vi "Get Measurement Variables from Recipe.vi"(8 "error in (no error)":errorcluster, 11 "Measurement in":refnum<class "Measurement.lvclass">) -> (0 "error out":errorcluster, 1 "Measurements":string[](array[string]), 2 "Power Measurements":string[](array[string]), 3 "Measurement Voltages":string[](array[string]))   [LabVIEW 2015, in "Measurement.lvclass"]
uses:
  Measurement.lvclass
  Test Class/Test Class.lvclass
  Classes/Application/Class/Application.lvclass
  Classes/Test Recipe/Class/Test Recipe.lvclass
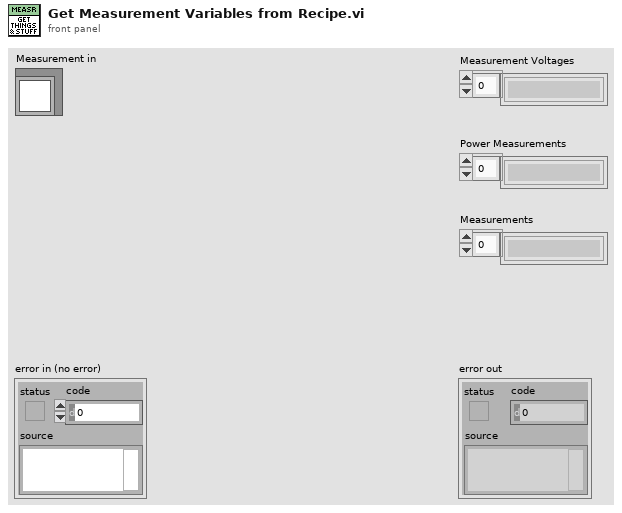
[diagram p1: front panel]
types:
  T1 = typedef "Application.lvlib/App Properties.lvclass/Class Properties -- Cluster.ctl" = cluster{"UUT Info":T2[], "Test Information":refnum<vi>, "Test Complete Event":refnum<user-event>, "Shop Floor System":refnum<class "Shop Floor System.lvclass">, "Gold Board":refnum<class "Golden Board.lvclass">, "Test Recipe":refnum<class "Test Recipe.lvclass">, "Instruments":refnum<class "Instrument.lvclass">[], "Mode":T3, "Test Results":cluster{"Pass":bool[], "Fail Codes":string[]}, "Station Config":refnum<class "Station Config.lvclass">}
  T2 = typedef "Application.lvlib/App Properties.lvclass/UUT Reference -- Cluster.ctl" = cluster{"Serial Number Reference":refnum<vi>, "Status Message Reference":refnum<vi>}
  T3 = typedef "Application.lvlib/Application.lvclass/Op Mode -- Enum.ctl" = u16
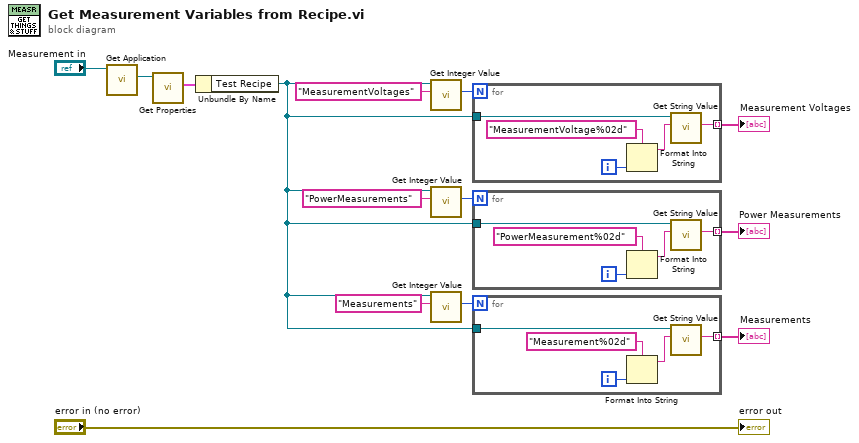
[diagram p0: block diagram]
diagram:
  n1 = call "Get Application.vi"("Test Class in"="Measurement in") -> ("Application.lvlib:Application.lvclass"=w12:refnum<class "Application.lvclass">)  [unwired: 9 in, 1 out]
  n2 = call "Get Properties.vi"("Acrobat Template in"=w12) -> ("Class Properties"=w11:T1)  [unwired: 8 in, 2 out]
  n3 = Unbundle By Name(w11) -> ("Test Recipe"=w2:refnum<class "Test Recipe.lvclass">)
  n4 = call "Get Integer Value.vi"("Name"="MeasurementVoltages", "Test Recipe in"=w2) -> ("Value"=w9:i32)  [unwired: 6 in, 3 out]
  n5 = call "Get Integer Value.vi"("Name"="PowerMeasurements", "Test Recipe in"=w2) -> ("Value"=w3:i32)  [unwired: 6 in, 3 out]
  n6 = call "Get Integer Value.vi"("Name"="Measurements", "Test Recipe in"=w2) -> ("Value"=w8:i32)  [unwired: 6 in, 3 out]
  n7 = for {
    N: w9 -> [_]
    tunnel: w2 -> [w19]
    tunnel: [w15] -> w6 mode=indexing
    i -> [w18]
    n8 = Format Into String(format string="MeasurementVoltage%02d", w18) -> (resulting string=w16:string)  [unwired: 2 in, 1 out]
    n9 = call "Get String Value.vi"("Name"=w16, "Test Recipe in"=w19) -> ("Value"=w15:string)  [unwired: 6 in, 3 out]
  }
  "Measurement Voltages" <- w6
  n10 = for {
    N: w3 -> [_]
    tunnel: w2 -> [w24]
    tunnel: [w20] -> w1 mode=indexing
    i -> [w23]
    n11 = Format Into String(format string="PowerMeasurement%02d", w23) -> (resulting string=w21:string)  [unwired: 2 in, 1 out]
    n12 = call "Get String Value.vi"("Name"=w21, "Test Recipe in"=w24) -> ("Value"=w20:string)  [unwired: 6 in, 3 out]
  }
  "Power Measurements" <- w1
  n13 = for {
    N: w8 -> [_]
    tunnel: w2 -> [w29]
    tunnel: [w25] -> w5 mode=indexing
    i -> [w28]
    n14 = Format Into String(format string="Measurement%02d", w28) -> (resulting string=w26:string)  [unwired: 2 in, 1 out]
    n15 = call "Get String Value.vi"("Name"=w26, "Test Recipe in"=w29) -> ("Value"=w25:string)  [unwired: 6 in, 3 out]
  }
  "Measurements" <- w5
  "error out" <- "error in (no error)"
